vi "niScope Fetch Array Measurement.vi"(0 "instrument handle":refnum<k15>, 1 "timeout":dbl=5.0 format="%.2f", 5 "channels":string="0", 7 "array measurement":T2=4000 items=["None"=4000, "Last Acq. Histogram"=4001, "Multi Acq. Voltage Histogram"=4004, "Multi Acq. Time Histogram"=4005, "Multi Acq. Average"=4016, "Polynomial Interpolation"=4011, "Array Integral"=4006, "Derivative"=4007, "Inverse"=4008, "Multiply Channels"=4012, "Add Channels"=4013, "Subtract Channels"=4014, "Divide Channels"=4015, "Array Offset"=4025, "Array Gain"=4026, "Hanning Window"=4009, "Flat Top Window"=4010, "Hamming Window"=4020, "Triangle Window"=4023, "Blackman Window"=4024, "FIR Windowed Filter"=4021, "Bessel IIR Filter"=4022, "Butterworth IIR Filter"=4017, "Chebyshev IIR Filter"=4018, "FFT Phase Spectrum"=4002, "FFT Amp. Spectrum (Volts RMS)"=4003, "FFT Amp. Spectrum (dB)"=4019], 11 "error in":errorcluster, 12 "meas waveform size":i32=-1) -> (4 "instrument handle out":refnum<k15>, 6 "meas wfm info":T1 {"reserved2" format="%.2f"; "reserved1" format="%.2f"; "offset" format="%^.3e"; "gain" format="%^.3e"; "xIncrement" format="%^.3e"; "relativeInitialX" format="%^.3e"; "absoluteInitialX" format="%^.3e"}, 10 "measWfm":dbl[](array[numeric]) format="%.2f", 15 "error out":errorcluster)   [LabVIEW 2013]
doc: "Obtains a waveform from the digitizer and returns the specified measurement voltage data for a single channel and record."
uses:
  <instrlib>/niScope/Controls/niScope array measurement.ctl
  niScope_32.dll
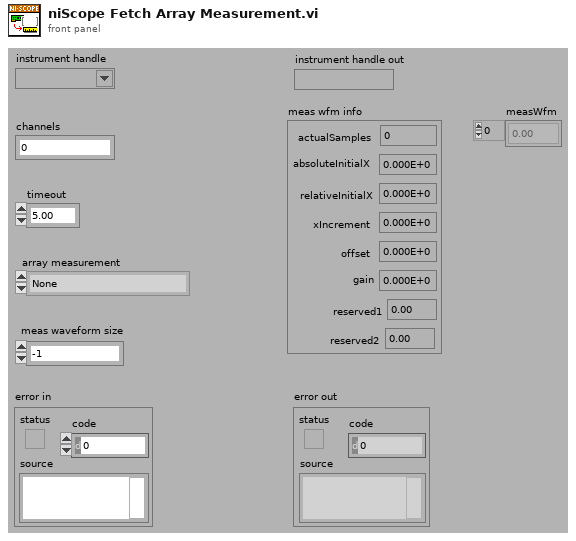
[diagram p1: front panel]
types:
  T1 = cluster{"actualSamples":i32, "absoluteInitialX":dbl, "relativeInitialX":dbl, "xIncrement":dbl, "offset":dbl, "gain":dbl, "reserved1":dbl, "reserved2":dbl}
  T2 = typedef "niScope array measurement.ctl" = i32
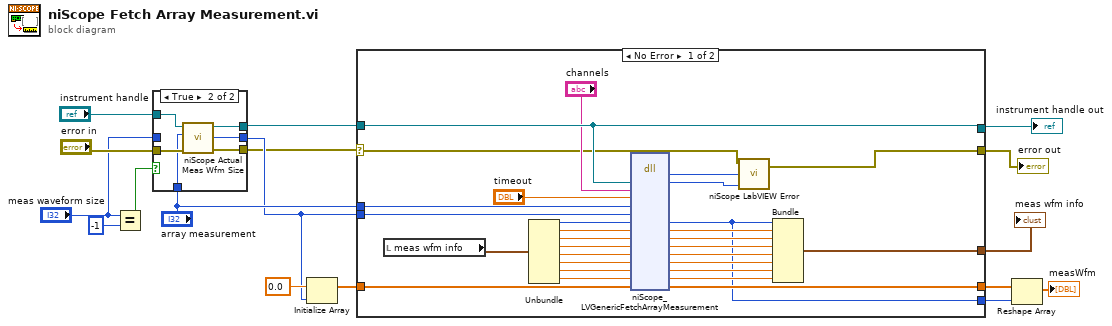
[diagram p0: block diagram]
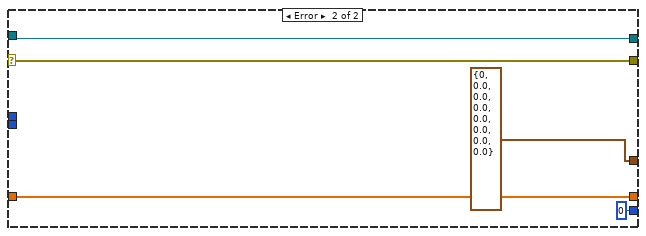
[diagram p3: hidden frame]
diagram:
  n1 = Equal?(x="meas waveform size", y=-1) -> (x = y?=w15:bool)
  n2 = case shown="True" w15 {
    tunnel: [w20 w26] -> w1
    tunnel: "error in" -> [w20 w25]
    tunnel: "instrument handle" -> [w19 w24]
    tunnel: [w19 w23] -> w10
    tunnel: [w18 w22] -> w5
    tunnel: "meas waveform size" -> [w18 _]
    tunnel: "array measurement" -> [_ w21]
    frame False {
    }
    frame True {
      n3 = call <instrlib>:"niScope Actual Meas Wfm Size.vi"("error in"=w25, "arrayMeasFunction"=w21, "instrument handle"=w24) -> ("error out"=w26:errorcluster, "meas wfm size"=w22:i32, "instrument handle out"=w23:refnum<k15>)  [unwired: 6 in]
    }
  }
  n4 = Initialize Array(0.0 ("Element Data"), w5) -> (w6:dbl[])
  n5 = case shown="No Error" w1 {
    selector: w1 -> [w27 w56]
    tunnel: [w55 w56] -> w17
    tunnel: w10 -> [w52 w60]
    tunnel: w5 -> [w45 _]
    tunnel: [w52 w60] -> w11
    tunnel: [w44 T1 {"actualSamples"=0, "absoluteInitialX"=0.0, "relativeInitialX"=0.0, "xIncrement"=0.0, "offset"=0.0, "gain"=0.0, "reserved1"=0.0, "reserved2"=0.0}] -> w8
    tunnel: "array measurement" -> [w39 _]
    tunnel: w6 -> [w42 w57]
    tunnel: [w29 w57] -> w3
    tunnel: [w28 0 ("actualSamples")] -> w2
    frame No Error {
      n6 = local read "meas wfm info"() -> (w38:T1)
      n7 = Unbundle(w38) -> ("actualSamples"=w37:i32, "absoluteInitialX"=w36:dbl, "relativeInitialX"=w35:dbl, "xIncrement"=w34:dbl, "offset"=w33:dbl, "gain"=w32:dbl, "reserved1"=w31:dbl, "reserved2"=w30:dbl)
      n8 = dll-call lib="niScope_*.*" fn="niScope_LVGenericFetchArrayMeasurement"("instrument handle"=w52, "channel"="channels", "timeout"="timeout", "arrayMeasFunction"=w39, "measWfmSize"=w45, "actualSamples"=w37, "absoluteInitialX"=w36, "relativeInitialX"=w35, "xIncrement"=w34, "offset"=w33, "gain"=w32, "reserved1"=w31, "reserved2"=w30, "measWfm"=w42) -> ("status"=w54:i32, "instrument handle"=w53:u32, "actualSamples"=w28:i32, "absoluteInitialX"=w46:dbl, "relativeInitialX"=w47:dbl, "xIncrement"=w48:dbl, "offset"=w49:dbl, "gain"=w50:dbl, "reserved1"=w41:dbl, "reserved2"=w40:dbl, "measWfm"=w29:dbl[])  [unwired: 7 in, 2 out]
      n9 = call <instrlib>:"niScope LabVIEW Error.vi"("instrument handle"=w53, "niScope error code (0)"=w54, "error in (no error)"=w27) -> ("error out"=w55:errorcluster)  [unwired: 2 in]
      n10 = Bundle("actualSamples"=w28, "absoluteInitialX"=w46, "relativeInitialX"=w47, "xIncrement"=w48, "offset"=w49, "gain"=w50, "reserved1"=w41, "reserved2"=w40) -> (w44:T1)  [unwired: 1 in]
    }
    frame Error {
    }
  }
  "error out" <- w17
  "instrument handle out" <- w11
  "meas wfm info" <- w8
  n11 = Reshape Array(w3, w2) -> (→"measWfm":dbl[])
